vi "get_fq_for_cz.vi"(11 "lc_num":string) -> (0 "zc_luodi_num":string, 1 "syren":string, 2 "fqren":string, 3 "fqbumen":string, 4 "error":errorcluster caption="error out 4", 5 "zc_ini_state":string, 7 "fangshi":string)   [LabVIEW 2017, in "Lib_code.lvlib"]
uses:
  Lib_code.lvlib
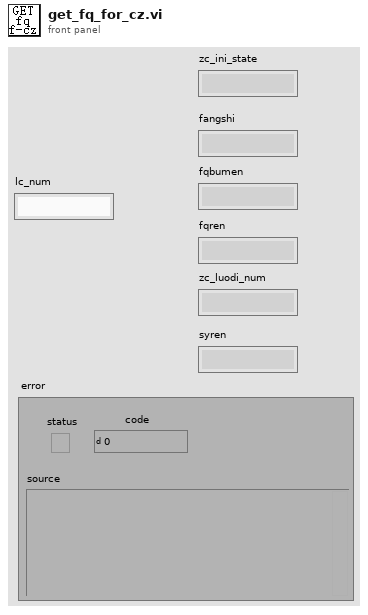
[diagram p1: front panel]
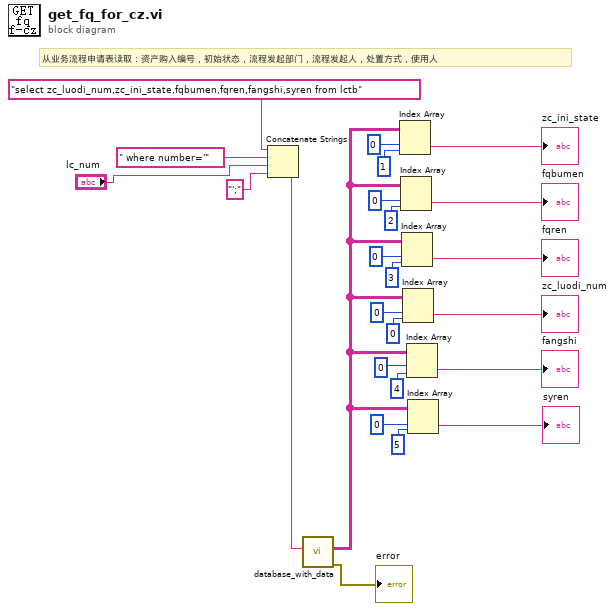
[diagram p0: block diagram]
diagram:
  # "从业务流程申请表读取：资产购入编号，初始状态，流程发起部门，流程发起人，处置方式，使用人"
  n1 = Concatenate Strings("select zc_luodi_num,zc_ini_state,fqbumen,fqren,fangshi,syren from lctb" ("Command Text"), " where number='" ("Command Text"), "lc_num", "';" ("字符串")) -> (w9:string)
  n2 = call "database_with_data.vi"("input"=w9) -> ("error"=→"error":errorcluster, "Data"=w1:string[][])  [unwired: 9 in]
  n3 = Index Array(array=w1, index (row)=0 ("索引 (行)"), index (col)=1 ("禁用的索引 (列)")) -> (element=→"zc_ini_state":string)
  n4 = Index Array(array=w1, index (row)=0 ("索引 (行)"), index (col)=2 ("禁用的索引 (列)")) -> (element=→"fqbumen":string)
  n5 = Index Array(array=w1, index (row)=0 ("索引 (行)"), index (col)=3 ("禁用的索引 (列)")) -> (element=→"fqren":string)
  n6 = Index Array(array=w1, index (row)=0 ("索引 (行)"), index (col)=0 ("禁用的索引 (列)")) -> (element=→"zc_luodi_num":string)
  n7 = Index Array(array=w1, index (row)=0 ("索引 (行)"), index (col)=4 ("禁用的索引 (列)")) -> (element=→"fangshi":string)
  n8 = Index Array(array=w1, index (row)=0 ("索引 (行)"), index (col)=5 ("禁用的索引 (列)")) -> (element=→"syren":string)
